vi "main_ctrl.vi"(8 "error in":errorcluster) -> (0 "error out":errorcluster caption="Error")   [LabVIEW 2013]
uses:
  <vilib>/Rock Robotics/WPI/DriverStation/WPI_DriverStationRobotMode2.ctl
  typedefs/fg_typedef.ctl
  typedefs/vision enable.ctl
  typedefs/subStates.ctl
  typedefs/singleUseSubstate.ctl
  <vilib>/Rock Robotics/WPI/Solenoid/WPI_SolenoidValue.ctl
  <vilib>/Rock Robotics/WPI/Compressor/WPI_CompressorGetSetRefNum.vi
  <vilib>/Rock Robotics/WPI/RobotDrive/WPI_RobotDriveGetSetRefNum.vi
  <vilib>/Rock Robotics/WPI/Solenoid/WPI_SolenoidSetEnum.vi
  <vilib>/Rock Robotics/WPI/RobotDrive/WPI_RobotDriveArcadeDrive_Standard(NoSaturation).vi
  typedefs/vision data.ctl
panel:
  out "Robot Mode":T1
  out "Vision SPI":u32
  out "Vision IPS":dbl
  out "Main IPS":dbl
  out "Main SPI":u32
  # "MAIN CONTROL"
  # "holds robot control code - dual parallel state machine"
  # "SPI: milliseconds per iteration\nIPS: iterations per second"
  # "need to incorporate cancel commands"
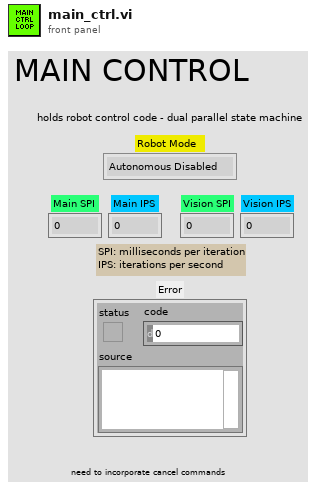
[diagram p1: front panel]
types:
  T1 = typedef "WPI_DriverStationRobotMode2.ctl" = enum16{"Autonomous Disabled", "Autonomous Enabled", "Teleop Disabled", "Teleop Enabled", "Timeout", "Finish", "Test Disabled", "Test Enabled"}
  T2 = typedef "vision data.ctl" = cluster{"x":dbl, "y":dbl, "area":dbl, "width":dbl, "height":dbl, "Hot Goal Present?":bool, "distance":dbl}
  T3 = typedef "vision enable.ctl" = enum16{"Enable", "Disable", "Stop"}
  T4 = typedef "fg_typedef.ctl" = enum16{"Get", "Set"}
  T5 = typedef "WPI_CameraDevRef.ctl" = cluster{"Camera Address":string, "CameraStatus":errorcluster, "Acquire Image Notifier":refnum<notifier>}
  T6 = typedef "IMAQ Image.ctl" = refnum<image>
  T7 = cluster{"Vision mSPI":u32, "Main mSPI":u32, "Dash mSPI":u32}
  T8 = typedef "WPI_RobotDriveDevRef.ctl" = cluster{"DevStatus":errorcluster, "Motors[]":T9[], "Square Inputs":bool, "Max Output":dbl, "Isochronous":bool}
  T9 = typedef "WPI_MotorControlDeviceRef.ctl" = cluster{"DeviceStatus":errorcluster, "Type":enum16{"PWM", "CAN"}, "PWM":cluster{"Digital Module":T10, "PWM Channel":T11, "DeadBand":T12}, "CAN":cluster{"Device Number":u8, "Control Mode":T13, "Semaphore":T14, "Max Vout":dbl}, "Invert":bool, "TransformRef":T15, "InvTransformRef":T15}
  T10 = typedef "FPGA_TypedefDigitalModule.ctl" = enum16{"Digital Module 1", "Digital Module 2"}
  T11 = typedef "FPGA_DIOPWMChannel.ctl" = enum8{"PWM 1", "PWM 2", "PWM 3", "PWM 4", "PWM 5", "PWM 6", "PWM 7", "PWM 8", "PWM 9", "PWM 10", "Invalid"}
  T12 = typedef "WPI_PWMDeadband.ctl" = cluster{"Name":string, "maxPositivePwm":i32, "minPositivePwm":i32, "centerPwm":i32, "maxNegativePwm":i32, "minNegativePwm":i32, "angularRange":u16}
  T13 = typedef "WPI_CANJaguar_ControlMode.ctl" = enum8{"Percent VBus", "Current", "Speed", "Position", "Voltage"}
  T14 = typedef "Semaphore RefNum" = refnum<k1>
  T15 = typedef "WPI_PWMTransform_ConPane.ctl" = refnum<vi>
  T16 = typedef "WPI_SolenoidDevRef.ctl" = cluster{"DevStatus":errorcluster, "Solenoid Module":T17, "Forward Solenoid Channel":T18, "Reverse Solenoid Channel":T18}
  T17 = typedef "FPGA_TypedefSolenoidModule.ctl" = enum16{"Solenoid Module 1", "Solenoid Module 2"}
  T18 = typedef "WPI_SolenoidChannel.ctl" = enum8{"Solenoid 1", "Solenoid 2", "Solenoid 3", "Solenoid 4", "Solenoid 5", "Solenoid 6", "Solenoid 7", "Solenoid 8", "Invalid"}
  T19 = typedef "WPI_CompressorDevRef.ctl" = cluster{"DevStatus":errorcluster, "DigitalInputDevRef":T20, "RelayDevRef":T22}
  T20 = typedef "WPI_DigitalInputDevRef.ctl" = cluster{"DevStatus":errorcluster, "DIO Channel":T21, "Digital Module":T10}
  T21 = typedef "FPGA_DIOChannel.ctl" = enum8{"DIO 1", "DIO 2", "DIO 3", "DIO 4", "DIO 5", "DIO 6", "DIO 7", "DIO 8", "DIO 9", "DIO 10", "DIO 11", "DIO 12", "DIO 13", "DIO 14", "Invalid"}
  T22 = typedef "WPI_RelayDevRef.ctl" = cluster{"DevStatus":errorcluster, "Relay Channel":T23, "Digital Module":T10, "Relay Direction":T24}
  T23 = typedef "FPGA_DIORelayChannel.ctl" = enum8{"Relay 1", "Relay 2", "Relay 3", "Relay 4", "Relay 5", "Relay 6", "Relay 7", "Relay 8", "Invalid"}
  T24 = typedef "WPI_RelayDirection.ctl" = enum16{"Both directions", "Forward only", "Reverse only"}
  T25 = typedef "WPI_SolenoidValue.ctl" = enum16{"Off", "On", "Forward", "Reverse"}
  T26 = typedef "singleUseSubstate.ctl" = enum16{"null", "wait", "shift high", "shift low"}
  T27 = typedef "WPI_DriverStationDerivedRobotMode.ctl" = enum16{"Init", "Execute", "Stop"}
  T28 = typedef "subStates.ctl" = enum16{"null", "wait", "driver control", "auto", "manual override", "hold position", "rotate", "pickup", "pass", "load", "goto shoot", "shoot", "cancel", "end"}
  T29 = typedef "Loop 2 Datatype.ctl" = cluster{"State":T28, "Waiting Loop":i32, "State to Wait For":i32, "Loop ID":i32, "Exit Value":i32, "Joystick Y":dbl, "Tune Speed":dbl}
  T30 = typedef "Loop 1 Datatype.ctl" = cluster{"State":T28, "Waiting Loop":i32, "State to Wait For":i32, "Loop ID":i32, "Exit Value":i32}
  T31 = typedef "Loop 3 Datatype.ctl" = cluster{"State":T28, "Waiting Loop":i32, "State to Wait For":i32, "Loop ID":i32, "Exit Value":i32, "Joystick Y":dbl, "Joystick Z":dbl}
  T32 = typedef "Loop 0 Datatype.ctl" = cluster{"State":T28, "Waiting Loop":i32, "State to Wait For":i32, "Loop ID":i32, "Exit Value":i32, "X Axis":dbl, "Y Axis":dbl, "Z Axis":dbl}
  T33 = typedef "Loop 4 Datatype.ctl" = cluster{"State":T28, "Waiting Loop":i32, "State to Wait For":i32, "Loop ID":i32, "Exit Value":i32}
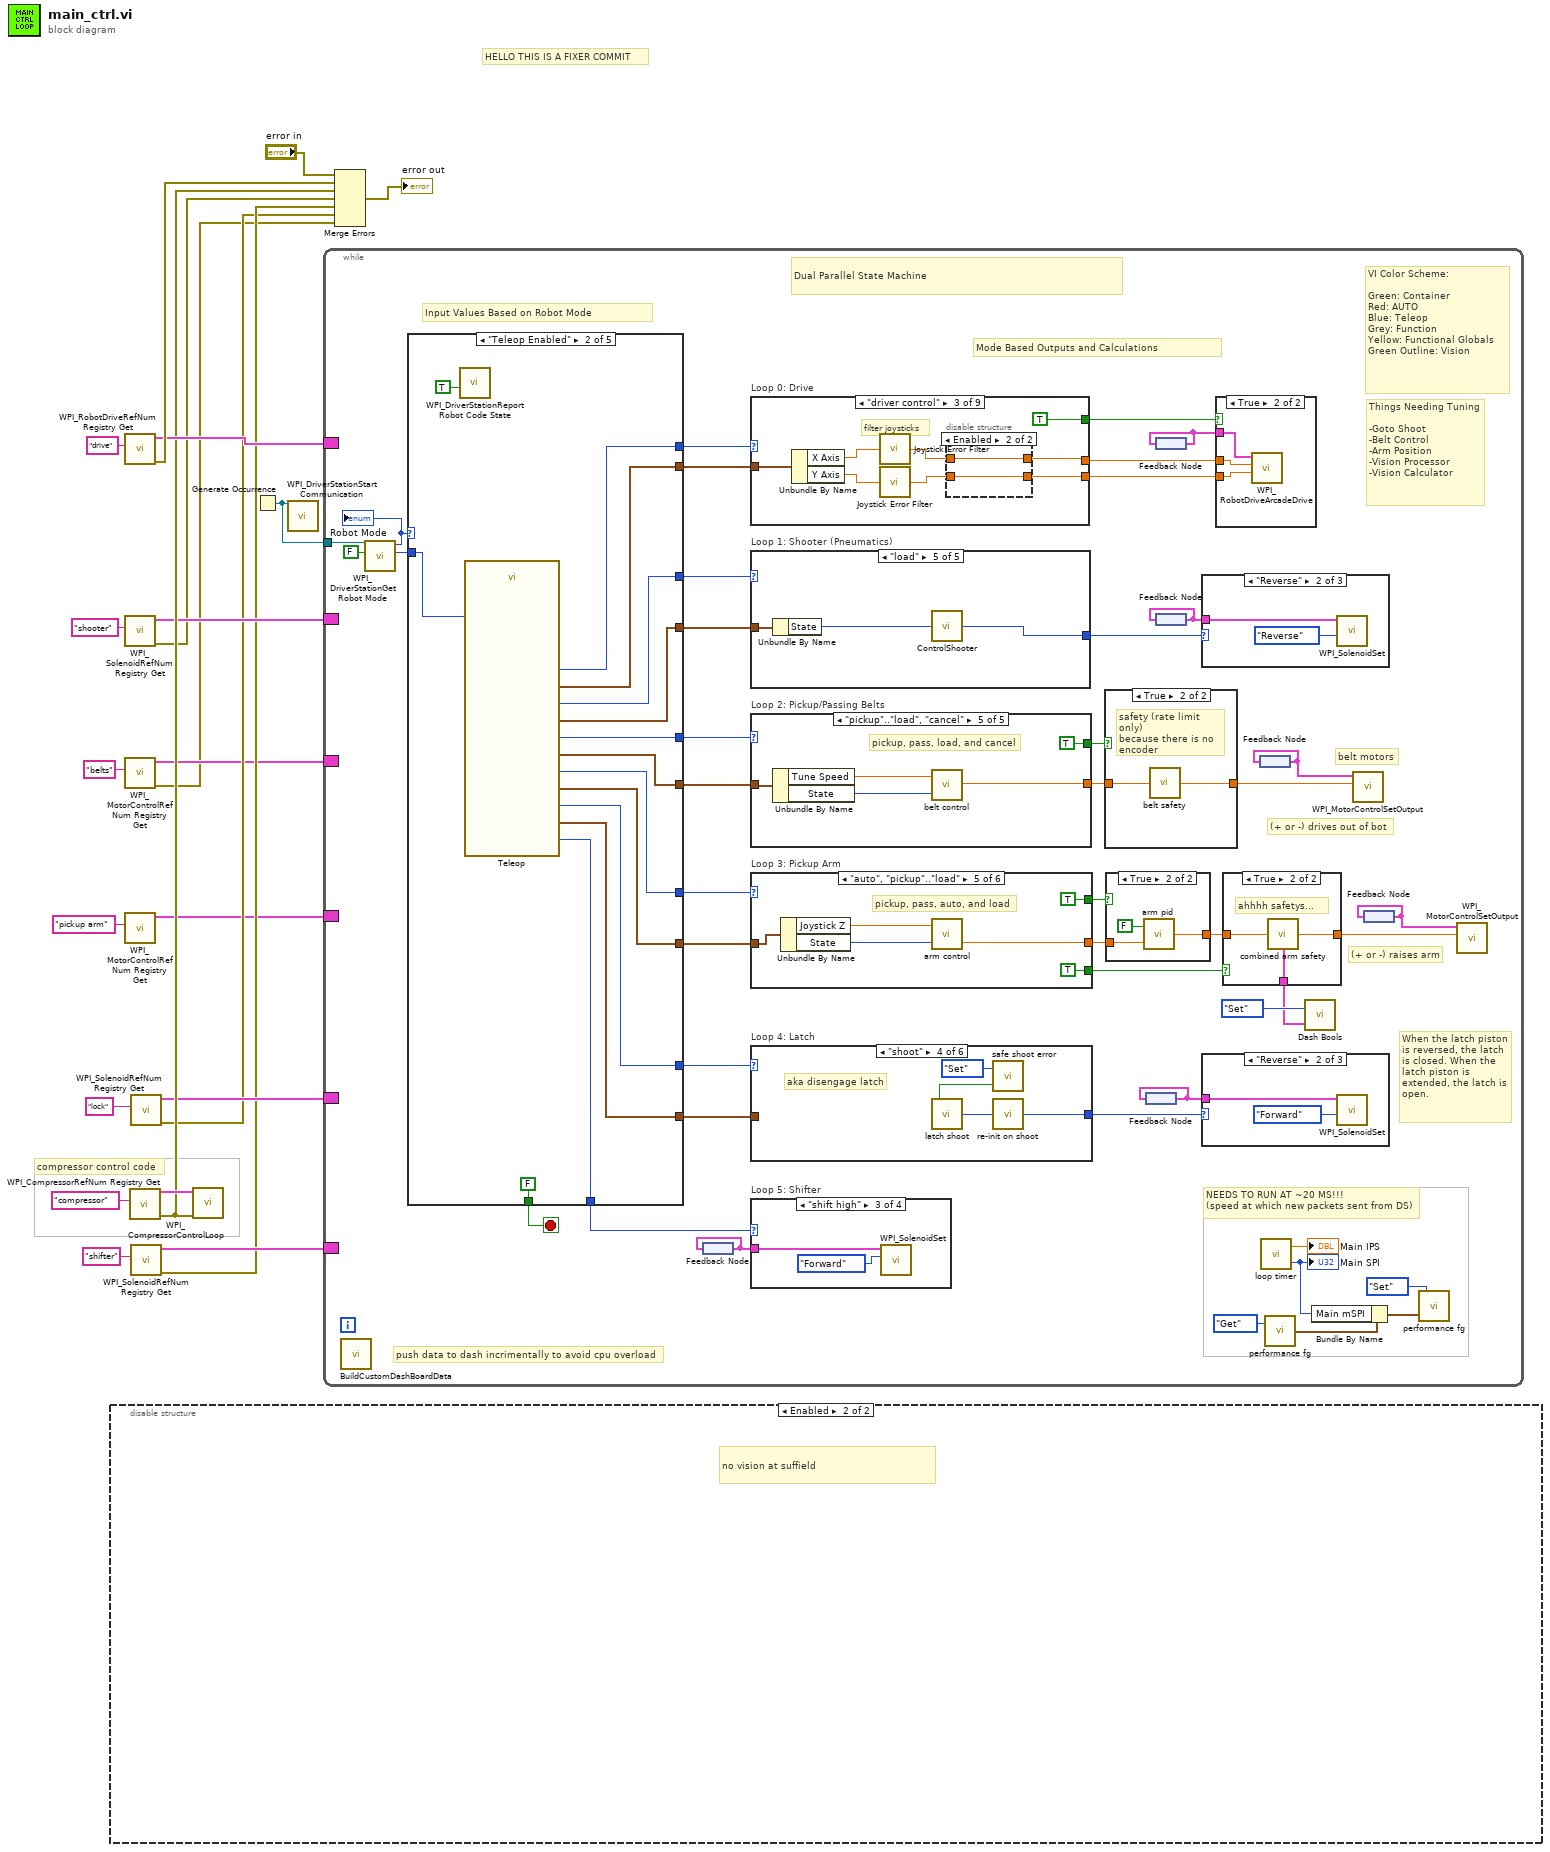
[diagram p0: block diagram]
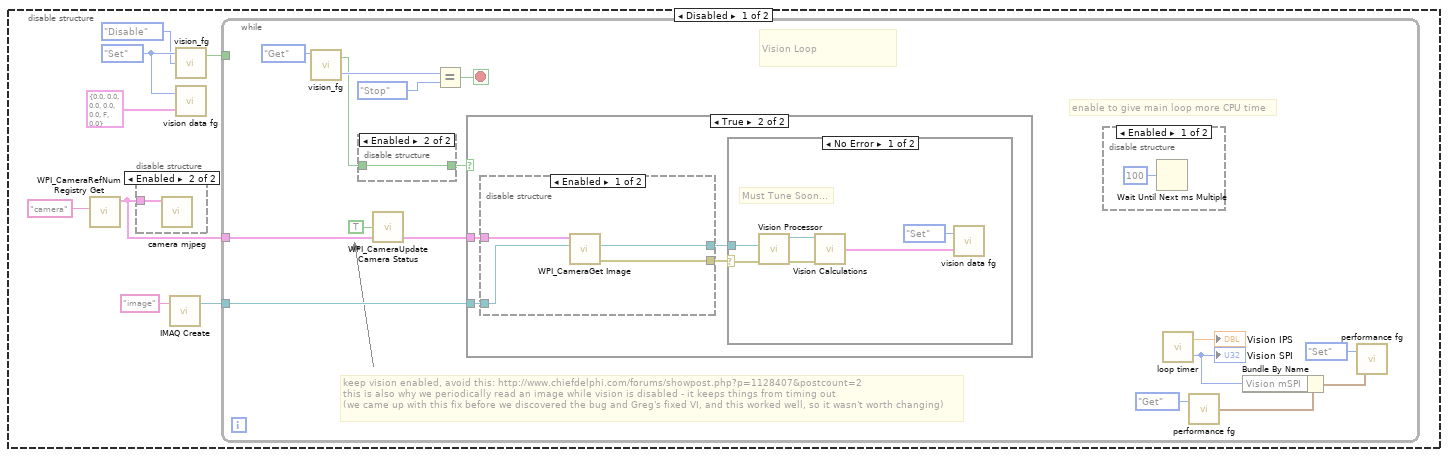
[diagram p2: hidden frame]
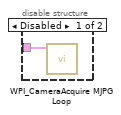
[diagram p3: hidden frame]
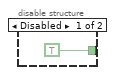
[diagram p4: hidden frame]
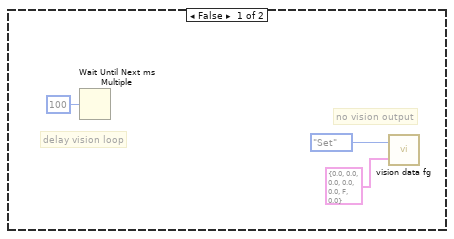
[diagram p6: hidden frame]
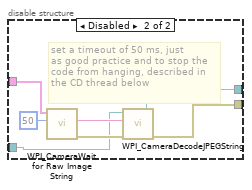
[diagram p8: hidden frame]
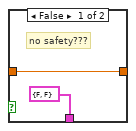
[diagram p10: hidden frame]
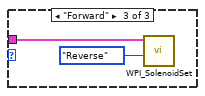
[diagram p13: hidden frame]
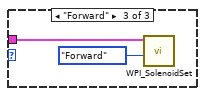
[diagram p15: hidden frame]
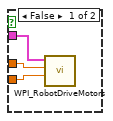
[diagram p16: hidden frame]
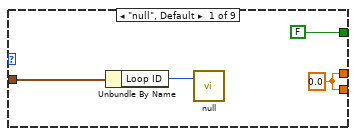
[diagram p17: hidden frame]
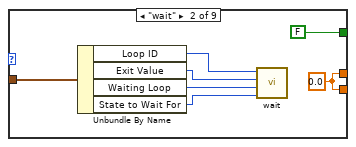
[diagram p18: hidden frame]
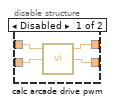
[diagram p19: hidden frame]
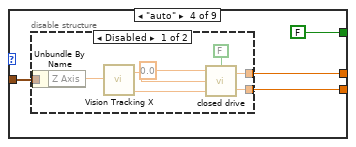
[diagram p20: hidden frame]
diagram:
  # "compressor control code"
  # "HELLO THIS IS A FIXER COMMIT"
  n1 = disable-structure shown="Enabled" {
    frame Disabled {
      w29 = fg_typedef."Set" ("Enum")
      n2 = call <vilib>:"WPI_CameraRefNum Registry Get.vi"("refnum name"="camera") -> ("CameraDevRef"=w26:T5)  [unwired: 9 in, 1 out]
      n3 = disable-structure shown="Enabled" {
        disable-tunnel: w26 -> [w32 w33]
        frame Disabled {
          n4 = call <vilib>:"WPI_CameraAcquire MJPG Loop.vi"("CameraDevRef"=w32) -> ()  [unwired: 11 in]
        }
        frame Enabled {
          n5 = call "camera mjpeg.vi"("CameraDevRef"=w33) -> ()  [unwired: 11 in]
        }
      }
      n6 = call "IMAQ Create"("Image Name"="image") -> ("New Image"=w31:T6)  [unwired: 4 in, 1 out]
      n7 = call "vision_fg.vi"("Action"=vision_enable."Disable", "Menu"=w29) -> ("Enabled?"=w30:bool)  [unwired: 1 in, 1 out]
      n8 = call "vision data fg.vi"("Input"=T2 {"x"=0.0, "y"=0.0, "area"=0.0, "width"=0.0, "height"=0.0, "Hot Goal Present?"=FALSE, "distance"=0.0} ("Cluster"), "Menu"=w29) -> ()  [unwired: 1 out]
      n9 = while {
        tunnel: w31 -> [w48]
        tunnel: w26 -> [w47]
        tunnel: w30 -> [_]
        stop <- w49 stop-if-true
        # "keep vision enabled, avoid this: http://www.chiefdelphi.com/forums/showpost.php?p=1128407&postcount=2\nthis is also why we periodically read an image while vision is disabled - it keeps things from timing out\n(we came up with this fix before we discovered the bug and Greg's fixed VI, and this worked well, so it wasn't worth changing)"
        # "enable to give main loop more CPU time"
        # "Vision Loop"
        n10 = call "vision_fg.vi"("Menu"=fg_typedef."Get" ("Enum")) -> ("State Out"=w43:T3, "Enabled?"=w34:bool)  [unwired: 2 in]
        n11 = disable-structure shown="Enabled" {
          disable-tunnel: [TRUE w51] -> w35
          disable-tunnel: w34 -> [_ w51]
          frame Disabled {
          }
          frame Enabled {
          }
        }
        n12 = call <vilib>:"WPI_CameraUpdate Camera Status.vi"("CameraDevRef In"=w47, "Enable Vision"=TRUE) -> ("CameraDevRef Out"=w46:T5)  [unwired: 3 in]
        n13 = Equal?(x=w43, y=vision_enable."Stop") -> (x = y?=w49:bool)
        n14 = case shown="True" w35 {
          tunnel: w48 -> [_ w59]
          tunnel: w46 -> [_ w58]
          frame False {
            # "no vision output"
            # "delay vision loop"
            n15 = Wait Until Next ms Multiple(millisecond multiple=u32 100) -> ()  [unwired: 1 out]
            n16 = call "vision data fg.vi"("Input"=T2 {"x"=0.0, "y"=0.0, "area"=0.0, "width"=0.0, "height"=0.0, "Hot Goal Present?"=FALSE, "distance"=0.0} ("Cluster"), "Menu"=fg_typedef."Set" ("Enum")) -> ()  [unwired: 1 out]
          }
          frame True {
            n17 = disable-structure shown="Enabled" {
              disable-tunnel: w59 -> [w68 w72]
              disable-tunnel: w58 -> [w69 w74]
              disable-tunnel: [w67 w71] -> w57
              disable-tunnel: [w66 w70] -> w56
              frame Enabled {
                n18 = call <vilib>:"WPI_CameraGet Image.vi"("Image"=w68, "CameraDevRef"=w69) -> ("error out"=w66:errorcluster, "Image Out"=w67:T6)  [unwired: 7 in, 1 out]
              }
              frame Disabled {
                # "set a timeout of 50 ms, just\nas good practice and to stop the \ncode from hanging, described in \nthe CD thread below"
                n19 = call <vilib>:"WPI_CameraWait for Raw Image String.vi"("Timeout in ms (-1)"=50, "CameraDevRef"=w74) -> ("error out"=w76:errorcluster, "String"=w75:string)  [unwired: 3 in, 5 out]
                n20 = call <vilib>:"WPI_CameraDecodeJPEGString.vi"("error in"=w76, "Compressed Image"=w75, "Image In"=w72) -> ("error out"=w70:errorcluster, "Image Out"=w71:T6)  [unwired: 3 out]
              }
            }
            n21 = case shown="No Error" w56 {
              selector: w56 -> [w64 _]
              tunnel: w57 -> [w63 _]
              frame No Error {
                # "Must Tune Soon..."
                n22 = call "Vision Processor.vi"("error in"=w64, "Image In"=w63) -> ("error out"=w61:errorcluster, "Image Out"=w62:T6)  [unwired: 5 in]
                n23 = call "Vision Calculations.vi"("Image In"=w62, "error in"=w61) -> ("Vision Data"=w60:T2)  [unwired: 3 in]
                n24 = call "vision data fg.vi"("Input"=w60, "Menu"=fg_typedef."Set" ("Enum")) -> ()  [unwired: 1 out]
              }
              frame Error {
              }
            }
          }
        }
        n25 = disable-structure shown="Enabled" {
          frame Enabled {
            n26 = Wait Until Next ms Multiple(millisecond multiple=u32 100) -> ()  [unwired: 1 out]
          }
          frame Disabled {
          }
        }
        n27 = call "loop timer.vi"() -> ("IPS"=→"Vision IPS":dbl, "SPI"=w41:u32)  [unwired: 1 in]
        "Vision SPI" <- w41
        n28 = call "performance fg.vi"("Menu"=fg_typedef."Get") -> ("Output"=w39:T7)  [unwired: 1 in]
        n29 = Bundle By Name(cluster=w39, "Vision mSPI"=w41) -> (w38:T7)
        n30 = call "performance fg.vi"("Input"=w38, "Menu"=fg_typedef."Set") -> ()  [unwired: 1 out]
      }
    }
    frame Enabled {
      # "no vision at suffield"
    }
  }
  n31 = call <vilib>:"WPI_RobotDriveRefNum Registry Get.vi"("refnum name"="drive") -> ("error out"=w20:errorcluster, "RobotDriveDevRef"=w18:T8)  [unwired: 9 in]
  n32 = call <vilib>:"WPI_SolenoidRefNum Registry Get.vi"("refnum name"="shooter") -> ("error out"=w7:errorcluster, "SolenoidDevRef"=w11:T16)  [unwired: 9 in]
  n33 = call <vilib>:"WPI_MotorControlRefNum Registry Get.vi"("refnum name"="belts") -> ("error out"=w3:errorcluster, "MotorControlDevRef"=w5:T9)  [unwired: 9 in]
  n34 = call <vilib>:"WPI_MotorControlRefNum Registry Get.vi"("refnum name"="pickup arm") -> ("MotorControlDevRef"=w1:T9)  [unwired: 9 in, 1 out]
  n35 = call <vilib>:"WPI_CompressorRefNum Registry Get.vi"("refnum name"="compressor") -> ("error out"=w14:errorcluster, "CompressorDevRef"=w17:T19)  [unwired: 9 in]
  n36 = call <vilib>:"WPI_SolenoidRefNum Registry Get.vi"("refnum name"="lock") -> ("error out"=w6:errorcluster, "SolenoidDevRef"=w9:T16)  [unwired: 9 in]
  n37 = call <vilib>:"WPI_SolenoidRefNum Registry Get.vi"("refnum name"="shifter") -> ("error out"=w8:errorcluster, "SolenoidDevRef"=w16:T16)  [unwired: 9 in]
  n38 = call <vilib>:"WPI_CompressorControlLoop.vi"("error in (no error)"=w14, "CompressorDevRef"=w17) -> ()  [unwired: 10 in]
  n39 = Generate Occurrence() -> (w13:refnum<k4>)
  n40 = call <vilib>:"WPI_DriverStationStart Communication.vi"("occurrence"=w13) -> ()  [unwired: 11 in]
  n41 = while {
    tunnel: w13 -> [w95]
    border: w18 -> [_]
    border: w16 -> [_]
    border: w11 -> [_]
    border: w9 -> [_]
    border: w5 -> [_]
    border: w1 -> [_]
    stop <- w116 stop-if-true
    # "When the latch piston\nis reversed, the latch\nis closed. When the\nlatch piston is\nextended, the latch is\nopen."
    # "push data to dash incrimentally to avoid cpu overload"
    # "Things Needing Tuning\n\n-Goto Shoot\n-Belt Control\n-Arm Position\n-Vision Processor\n-Vision Calculator"
    # "(+ or -) raises arm"
    # "(+ or -) drives out of bot"
    # "belt motors"
    # "VI Color Scheme:\n\nGreen: Container\nRed: AUTO\nBlue: Teleop\nGrey: Function\nYellow: Functional Globals\nGreen Outline: Vision"
    # "Input Values Based on Robot Mode"
    # "Mode Based Outputs and Calculations"
    # "NEEDS TO RUN AT ~20 MS!!!\n(speed at which new packets sent from DS)"
    # "Dual Parallel State Machine"
    n42 = call "BuildCustomDashBoardData.vi"() -> ()  [unwired: 12 in]
    n43 = call <vilib>:"WPI_DriverStationGet Robot Mode.vi"("Finish"=FALSE, "DS Occurrence"=w95) -> ("Call Context"=w94:T27, "Robot Mode"=w93:T1)  [unwired: 8 out]
    "Robot Mode" <- w93
    n44 = case shown="\"Teleop Enabled\"" w93 {
      tunnel: [w312 w329 w331 w337 w343] -> w97
      tunnel: w94 -> [w303 w325 _ _ _]
      tunnel: [w310 w328 w331 w337 w343] -> w118
      tunnel: [w304 w326 singleUseSubstate."null" ("SubState 5") singleUseSubstate."null" ("SubState 5") singleUseSubstate."null" ("SubState 5")] -> w117
      tunnel: [FALSE FALSE FALSE FALSE TRUE] -> w116
      tunnel: [w314 w324 w331 w337 w343] -> w109
      tunnel: [w313 w323 _ _ _] -> w110
      tunnel: [w311 w322 _ _ _] -> w108
      tunnel: [w309 w321 _ _ _] -> w107
      tunnel: [w307 w320 _ _ _] -> w105
      tunnel: [w305 w319 _ _ _] -> w104
      tunnel: [w306 w318 w331 w337 w343] -> w103
      tunnel: [w308 w317 w331 w337 w343] -> w102
      frame "Autonomous Enabled" {
        n45 = call <vilib>:"WPI_DriverStationReport Robot Code State.vi"("Autonomous"=TRUE) -> ()  [unwired: 10 in, 1 out]
        n46 = call "Autonomous.vi"("Call Context"=w303) -> ("SubState 2"=w310:T28, "Loop 2 Data"=w309:T29, "SubState 1"=w312:T28, "Loop 1 Data"=w311:T30, "Loop 3 Data"=w307:T31, "SubState 0"=w314:T28, "SubState 3"=w308:T28, "Loop 0 Data"=w313:T32, "Loop 4 Data"=w305:T33, "SubState 4"=w306:T28, "SubState 5"=w304:T26)
      }
      frame "Teleop Enabled" {
        n47 = call <vilib>:"WPI_DriverStationReport Robot Code State.vi"("TeleOp"=TRUE) -> ()  [unwired: 10 in, 1 out]
        n48 = call "Teleop.vi"("Call Context"=w325) -> ("SubState 3"=w317:T28, "SubState 4"=w318:T28, "SubState 5"=w326:T26, "Loop 3 Data"=w320:T31, "Loop 4 Data"=w319:T33, "SubState 0"=w324:T28, "Loop 1 Data"=w322:T30, "Loop 0 Data"=w323:T32, "SubState 1"=w329:T28, "Loop 2 Data"=w321:T29, "SubState 2"=w328:T28)  [unwired: 8 in]
      }
      frame "Autonomous Disabled", "Teleop Disabled", "Timeout" {
        w331 = subStates."null" ("SubState 0")
        # "set all loops to null"
        # "make sure to disable vision\nwe don't need it here"
        # "robot disabled, timeout"
        n49 = call <vilib>:"WPI_DriverStationReport Robot Code State.vi"("Disabled"=TRUE) -> ()  [unwired: 10 in, 1 out]
        n50 = call "vision_fg.vi"("Action"=vision_enable."Disable", "Menu"=fg_typedef."Set") -> ()  [unwired: 1 in, 2 out]
      }
      frame "Test Disabled", "Test Enabled" {
        w337 = subStates."null" ("SubState 0")
        # "set all loops to null"
        # "make sure to disable vision\nwe don't need it here"
        # "test, unused"
        n51 = call <vilib>:"WPI_DriverStationReport Robot Code State.vi"("Test"=TRUE) -> ()  [unwired: 10 in, 1 out]
        n52 = call "vision_fg.vi"("Action"=vision_enable."Disable", "Menu"=fg_typedef."Set") -> ()  [unwired: 1 in, 2 out]
      }
      frame "Finish" {
        w343 = subStates."end"  # Stop All Loops
        # "stop the while loop"
        # "stop DS comms"
        # "stop vision loop"
        n53 = call <vilib>:"WPI_DriverStationStop Communication.vi"("StopCommunication"=TRUE) -> ()  [unwired: 10 in, 1 out]
        n54 = call "vision_fg.vi"("Action"=vision_enable."Stop", "Menu"=fg_typedef."Set") -> ()  [unwired: 1 in, 2 out]
      }
    }
    n55 = feedback #1() -> (w106:T16)
    n56 = feedback-in #1(w106) -> ()
    n57 = case "Loop 0: Drive" shown="\"driver control\"" w109 {
      tunnel: w110 -> [w148 w152 w164 w171 w188 w195 _ _ w211]
      tunnel: [w146 w150 w162 w173 w185 w197 w200 w205 w207] -> w100
      tunnel: [w146 w150 w161 w172 w184 w196 w199 w205 w206] -> w99
      tunnel: [FALSE FALSE TRUE FALSE FALSE FALSE FALSE FALSE FALSE] -> w101
      frame "null", Default {
        w146 = 0.0 ("X Axis")
        n58 = Unbundle By Name(w148) -> ("Loop ID"=w149:i32)
        n59 = call "null.vi"("This Loop ID"=w149) -> ()  [unwired: 2 in]
      }
      frame "wait" {
        w150 = 0.0 ("X Axis")
        n60 = Unbundle By Name(w152) -> ("Loop ID"=w156:i32, "Exit Value"=w155:i32, "Waiting Loop"=w154:i32, "State to Wait For"=w153:i32)
        n61 = call "wait.vi"("State to wait for"=w153, "Waiting Loop ID"=w154, "time (ms)"=w155, "Current Loop ID"=w156) -> ()  [unwired: 1 out]
      }
      frame "driver control" {
        # "filter joysticks"
        n62 = Unbundle By Name(w164) -> ("X Axis"=w157:dbl, "Y Axis"=w160:dbl)
        n63 = call "Joystick Error Filter.vi"("Axis"=w157) -> ("Filtered Axis"=w158:dbl)
        n64 = call "Joystick Error Filter.vi"("Axis"=w160) -> ("Filtered Axis"=w159:dbl)
        n65 = disable-structure shown="Enabled" {
          disable-tunnel: w158 -> [w168 w170]
          disable-tunnel: w159 -> [w167 w169]
          disable-tunnel: [w166 w170] -> w162
          disable-tunnel: [w165 w169] -> w161
          frame Disabled {
            n66 = call "calc arcade drive pwm.vi"("Y axis value"=w167, "X axis value"=w168) -> ("Right Speed"=w165:dbl, "Left Speed"=w166:dbl)  [unwired: 1 in, 1 out]
          }
          frame Enabled {
          }
        }
      }
      frame "auto" {
        n67 = disable-structure shown="Disabled" {
          disable-tunnel: [w182 _] -> w173
          disable-tunnel: [w181 _] -> w172
          disable-tunnel: w171 -> [w177 _]
          frame Disabled {
            n68 = Unbundle By Name(w177) -> ("Z Axis"=w175:dbl)
            n69 = call "Vision Tracking X.vi"("Tweak"=w175) -> ("right speed"=w176:dbl, "left speed"=w179:dbl)
            n70 = call "closed drive.vi"("Acrade Drive?"=FALSE, "Y axis value (Left)"=w179, "X axis value (Right)"=w176, "Threshold (.4)"=0.0 ("Threshold")) -> ("right"=w181:dbl, "left"=w182:dbl)
          }
          frame Enabled {
            # "rotates toward target"
            # "not in use this year"
          }
        }
      }
      frame "hold position" {
        n71 = Unbundle By Name(w188) -> ("X Axis"=w187:dbl, "Y Axis"=w186:dbl)
        n72 = call "closed drive.vi"("Acrade Drive?"=TRUE, "Y axis value (Left)"=w186, "X axis value (Right)"=w187) -> ("right"=w184:dbl, "left"=w185:dbl)  [unwired: 1 in]
      }
      frame "rotate" {
        # "use these to carry actual information because this is\nfor autonomous only so there will not be joystick input"
        n73 = Unbundle By Name(w195) -> ("X Axis"=w194:dbl, "Y Axis"=w193:dbl)
        n74 = call "rotate.vi"("Angle"=w194, "Rate"=w193) -> ("finished?"=w190:bool, "left speed"=w197:dbl, "right speed"=w196:dbl)
        n75 = call "states FG.vi"("exit in"=w190, "menu (get)"=enum16{"set", "get"}."set", "Loop ID"=0) -> ()  [unwired: 5 in, 4 out]
      }
      frame "goto shoot" {
        # "consider implimenting closed hold with drive"
        n76 = call "vision data fg.vi"("Menu"=fg_typedef."Get") -> ("Output"=w201:T2)  [unwired: 1 in]
        n77 = call "goto location.vi"("Image Data"=w201) -> ("left speed"=w200:dbl, "right speed"=w199:dbl)
      }
      frame "end" {
        w205 = 0.0 ("X Axis")
      }
      frame "manual override" {
        n78 = Unbundle By Name(w211) -> ("X Axis"=w210:dbl, "Y Axis"=w209:dbl)
        n79 = expression code="x/2"(w210) -> (w207:dbl)
        n80 = expression code="x/2"(w209) -> (w206:dbl)
      }
    }
    n81 = case "Loop 1: Shooter (Pneumatics)" shown="\"load\"" w97 {
      tunnel: w108 -> [w289 w292 _ _ w301]
      tunnel: [WPI_SolenoidValue."Off" ("Value") WPI_SolenoidValue."Off" ("Value") WPI_SolenoidValue."Off" ("Value") WPI_SolenoidValue."Off" ("Value") w299] -> w92
      frame "null", Default {
        n82 = Unbundle By Name(w289) -> ("Loop ID"=w290:i32)
        n83 = call "null.vi"("This Loop ID"=w290) -> ()  [unwired: 2 in]
      }
      frame "wait" {
        n84 = Unbundle By Name(w292) -> ("Loop ID"=w296:i32, "Exit Value"=w295:i32, "Waiting Loop"=w294:i32, "State to Wait For"=w293:i32)
        n85 = call "wait.vi"("State to wait for"=w293, "Waiting Loop ID"=w294, "time (ms)"=w295, "Current Loop ID"=w296) -> ()  [unwired: 1 out]
      }
      frame "driver control" {
      }
      frame "manual override" {
      }
      frame "load" {
        n86 = Unbundle By Name(w301) -> ("State"=w300:T28)
        n87 = call "ControlShooter.vi"("State"=w300) -> ("To Shooter\nSolenoid Loop"=w299:T25)
      }
    }
    n88 = case "Loop 2: Pickup/Passing Belts" shown="\"pickup\"..\"load\", \"cancel\"" w118 {
      tunnel: w107 -> [w267 w270 w278 w282 w287]
      tunnel: [0.0 ("output") 0.0 ("output") w276 w280 w284] -> w80
      tunnel: [FALSE FALSE TRUE FALSE TRUE] -> w81
      frame "null", Default {
        n89 = Unbundle By Name(w267) -> ("Loop ID"=w266:i32)
        n90 = call "null.vi"("This Loop ID"=w266) -> ()  [unwired: 2 in]
      }
      frame "wait" {
        n91 = Unbundle By Name(w270) -> ("Loop ID"=w274:i32, "Exit Value"=w273:i32, "Waiting Loop"=w272:i32, "State to Wait For"=w271:i32)
        n92 = call "wait.vi"("State to wait for"=w271, "Waiting Loop ID"=w272, "time (ms)"=w273, "Current Loop ID"=w274) -> ()  [unwired: 1 out]
      }
      frame "driver control" {
        n93 = Unbundle By Name(w278) -> ("Joystick Y"=w275:dbl)
        n94 = call "Joystick Error Filter.vi"("Axis"=w275) -> ("Filtered Axis"=w276:dbl)
      }
      frame "manual override" {
        n95 = Unbundle By Name(w282) -> ("Joystick Y"=w281:dbl)
        n96 = expression code="x/2"(w281) -> (w280:dbl)
      }
      frame "pickup".."load", "cancel" {
        # "pickup, pass, load, and cancel"
        n97 = Unbundle By Name(w287) -> ("Tune Speed"=w286:dbl, "State"=w285:T28)
        n98 = call "belt control.vi"("State"=w285, "Joystick Z"=w286) -> ("output"=w284:dbl)
      }
    }
    n99 = case "Loop 3: Pickup Arm" shown="\"auto\", \"pickup\"..\"load\"" w102 {
      tunnel: w105 -> [w232 w236 w244 w250 w256 _]
      tunnel: [FALSE FALSE FALSE FALSE TRUE TRUE] -> w86
      tunnel: [0.0 ("output") 0.0 ("output") w241 w248 w252 0.0 ("setpoint")] -> w85
      tunnel: [TRUE TRUE TRUE FALSE TRUE TRUE] -> w84
      frame "null", Default {
        n100 = Unbundle By Name(w232) -> ("Loop ID"=w231:i32)
        n101 = call "null.vi"("This Loop ID"=w231) -> ()  [unwired: 2 in]
      }
      frame "wait" {
        n102 = Unbundle By Name(w236) -> ("Loop ID"=w240:i32, "Exit Value"=w239:i32, "Waiting Loop"=w238:i32, "State to Wait For"=w237:i32)
        n103 = call "wait.vi"("State to wait for"=w237, "Waiting Loop ID"=w238, "time (ms)"=w239, "Current Loop ID"=w240) -> ()  [unwired: 1 out]
      }
      frame "driver control" {
        n104 = Unbundle By Name(w244) -> ("Joystick Y"=w242:dbl)
        n105 = call "Joystick Error Filter.vi"("Axis"=w242) -> ("Filtered Axis"=w241:dbl)
      }
      frame "manual override" {
        n106 = Unbundle By Name(w250) -> ("Joystick Y"=w249:dbl)
        n107 = expression code="x/2"(w249) -> (w248:dbl)
      }
      frame "auto", "pickup".."load" {
        # "pickup, pass, auto, and load"
        n108 = Unbundle By Name(w256) -> ("Joystick Z"=w254:dbl, "State"=w253:T28)
        n109 = call "arm control.vi"("State"=w253, "Z Axis (Tuning)"=w254) -> ("setpoint"=w252:dbl)
      }
      frame "hold position" {
        # "it just re-initalized, so 0 means don't move"
      }
    }
    n110 = case "Loop 4: Latch" shown="\"shoot\"" w103 {
      tunnel: w104 -> [w214 w216 _ _ _ _]
      tunnel: [WPI_SolenoidValue."Off" ("Value") WPI_SolenoidValue."Off" ("Value") WPI_SolenoidValue."Off" ("Value") w225 WPI_SolenoidValue."Forward" ("Value") WPI_SolenoidValue."Reverse" ("Value")] -> w89
      frame "null", Default {
        n111 = Unbundle By Name(w214) -> ("Loop ID"=w213:i32)
        n112 = call "null.vi"("This Loop ID"=w213) -> ()  [unwired: 2 in]
      }
      frame "wait" {
        n113 = Unbundle By Name(w216) -> ("Loop ID"=w220:i32, "Exit Value"=w219:i32, "Waiting Loop"=w218:i32, "State to Wait For"=w217:i32)
        n114 = call "wait.vi"("State to wait for"=w217, "Waiting Loop ID"=w218, "time (ms)"=w219, "Current Loop ID"=w220) -> ()  [unwired: 1 out]
      }
      frame "driver control" {
      }
      frame "shoot" {
        # "aka disengage latch"
        n115 = call "latch shoot.vi"() -> ("Latch"=w224:T25, "Met Requierments for shooting?"=w222:bool)
        n116 = call "safe shoot error.vi"("Can Shoot Safely?"=w222, "Menu"=fg_typedef."Set") -> ()  [unwired: 1 out]
        n117 = call "re-init on shoot.vi"("Relay Value"=w224) -> ("Value"=w225:T25)
      }
      frame "auto" {
        # "aka engage"
      }
      frame "manual override" {
        # "unsafely shoot"
      }
    }
    n118 = case "Loop 5: Shifter" shown="\"shift high\"" w117 {
      tunnel: w106 -> [_ _ w261 w262]
      frame "null", Default {
      }
      frame "wait" {
      }
      frame "shift high" {
        n119 = call-poly <vilib>:"WPI_SolenoidSet.vi"("Value"=WPI_SolenoidValue."Forward", "SolenoidDevRef"=w261) -> ()  [unwired: 8 in, 2 out]
      }
      frame "shift low" {
        n120 = call-poly <vilib>:"WPI_SolenoidSet.vi"("Value"=WPI_SolenoidValue."Reverse", "SolenoidDevRef"=w262) -> ()  [unwired: 8 in, 2 out]
      }
    }
    n121 = case shown="True" w81 {
      tunnel: w80 -> [w120 w122]
      tunnel: [w120 w121] -> w79
      frame False {
        # "no safety"
      }
      frame True {
        # "safety (rate limit only)\nbecause there is no \nencoder"
        n122 = call "belt safety.vi"("Input"=w122) -> ("Safe Output"=w121:dbl)
      }
    }
    n123 = case shown="True" w86 {
      tunnel: w85 -> [w128 w131]
      tunnel: [w128 w129] -> w83
      frame False {
        # "open loop"
      }
      frame True {
        n124 = call "arm pid.vi"("Setpoint"=w131, "Autotune?"=FALSE) -> ("Output"=w129:dbl)
      }
    }
    n125 = feedback #2() -> (w90:T16)
    n126 = feedback-in #2(w90) -> ()
    n127 = feedback #3() -> (w98:T8)
    n128 = feedback-in #3(w98) -> ()
    n129 = feedback #4() -> (w91:T16)
    n130 = feedback-in #4(w91) -> ()
    n131 = case shown="\"Reverse\"" w92 {
      tunnel: w91 -> [_ w136 w138]
      frame "Off", Default {
      }
      frame "Reverse" {
        n132 = call-poly <vilib>:"WPI_SolenoidSet.vi"("Value"=WPI_SolenoidValue."Reverse", "SolenoidDevRef"=w136) -> ()  [unwired: 8 in, 2 out]
      }
      frame "Forward" {
        n133 = call-poly <vilib>:"WPI_SolenoidSet.vi"("Value"=WPI_SolenoidValue."Forward", "SolenoidDevRef"=w138) -> ()  [unwired: 8 in, 2 out]
      }
    }
    n134 = case shown="\"Reverse\"" w89 {
      tunnel: w90 -> [_ w132 w134]
      frame "Off", Default {
      }
      frame "Reverse" {
        n135 = call-poly <vilib>:"WPI_SolenoidSet.vi"("Value"=WPI_SolenoidValue."Forward", "SolenoidDevRef"=w132) -> ()  [unwired: 8 in, 2 out]
      }
      frame "Forward" {
        n136 = call-poly <vilib>:"WPI_SolenoidSet.vi"("Value"=WPI_SolenoidValue."Reverse", "SolenoidDevRef"=w134) -> ()  [unwired: 8 in, 2 out]
      }
    }
    n137 = case shown="True" w101 {
      tunnel: w100 -> [w141 w145]
      tunnel: w99 -> [w140 w144]
      tunnel: w98 -> [w142 w143]
      frame False {
        n138 = call <vilib>:"WPI_RobotDriveMotors.vi"("RightSpeed"=w140, "LeftSpeed"=w141, "RobotDriveDevRef"=w142) -> ()  [unwired: 6 in, 3 out]
      }
      frame True {
        n139 = call-poly <vilib>:"WPI_RobotDriveArcadeDrive.vi"("Y axis value"=w144, "X axis value"=w145, "RobotDriveDevRef"=w143) -> ()  [unwired: 6 in, 3 out]
      }
    }
    n140 = case shown="True" w84 {
      tunnel: w83 -> [w124 w127]
      tunnel: [w124 w126] -> w82
      tunnel: [cluster{"Arm Safety":bool, "Arm Limit":bool} {"Arm Safety"=FALSE, "Arm Limit"=FALSE} ("Input") w125] -> w77
      frame False {
        # "no safety???"
      }
      frame True {
        # "ahhhh safetys..."
        n141 = call "combined arm safety.vi"("Input"=w127) -> ("Safe Output"=w126:dbl, "Safety"=w125:cluster{"Arm Safety":bool, "Arm Limit":bool})  [unwired: 13 in]
      }
    }
    n142 = feedback #5() -> (w88:T9)
    n143 = feedback-in #5(w88) -> ()
    n144 = call "loop timer.vi"() -> ("IPS"=→"Main IPS":dbl, "SPI"=w115:u32)  [unwired: 1 in]
    "Main SPI" <- w115
    n145 = call "performance fg.vi"("Menu"=fg_typedef."Get") -> ("Output"=w112:T7)  [unwired: 1 in]
    n146 = call "Dash Bools.vi"("Input"=w77, "Menu"=fg_typedef."Set") -> ()  [unwired: 1 out]
    n147 = Bundle By Name(cluster=w112, "Main mSPI"=w115) -> (w111:T7)
    n148 = call <vilib>:"WPI_MotorControlSetOutput.vi"("Output"=w79, "MotorControlDevRef"=w88) -> ()  [unwired: 7 in, 3 out]
    n149 = feedback #6() -> (w87:T9)
    n150 = feedback-in #6(w87) -> ()
    n151 = call "performance fg.vi"("Input"=w111, "Menu"=fg_typedef."Set") -> ()  [unwired: 1 out]
    n152 = call <vilib>:"WPI_MotorControlSetOutput.vi"("Output"=w82, "MotorControlDevRef"=w87) -> ()  [unwired: 7 in, 3 out]
  }
  n153 = Merge Errors("error in", w20, w14, w7, w8, w6, w3) -> (→"error out":errorcluster)
